vi "Layer Scan V1.vi"() -> ()   [LabVIEW 2024]
uses:
  <vilib>/DAQmx/create/channels.llb/DAQmx Create Channel (AO-Voltage-Basic).vi
  <vilib>/DAQmx/configure/timing.llb/DAQmx Timing (Sample Clock).vi
  <vilib>/DAQmx/configure/trigger.llb/DAQmx Start Trigger (Digital Edge).vi
  <vilib>/measure/NI_MAPro.lvlib
  <vilib>/express/express analysis/Spectral/XNode/ExpressSpectralMeasurementsBlockNode.xnode
  <vilib>/express/express analysis/Spectral/Block/exnSpectralBlock spectral measurements RMS poly.vi
  <vilib>/measure/NI_MABase.lvlib
  <vilib>/DAQmx/write.llb/DAQmx Write (Analog 2D DBL NChan NSamp).vi
  <vilib>/DAQmx/write.llb/DAQmx Write (Analog DBL 1Chan 1Samp).vi
  <vilib>/DAQmx/create/channels.llb/DAQmx Create Channel (AI-Voltage-Basic).vi
  <vilib>/DAQmx/write.llb/DAQmx Write (Analog 1D DBL NChan 1Samp).vi
  <vilib>/express/express analysis/Spectral/Block/exnSpectralBlock spectral measurements RMS WFM.vi
  <vilib>/DAQmx/read.llb/DAQmx Read (Analog DBL 1Chan 1Samp).vi
panel:
  out "Array":dbl[][](array[numeric])
  out "scan position #":i32
  in  "Laser Vibrometer CDAQ Channel":tag
  out "Waveform Graph":waveform(dbl)(graph)
  in  "Scan area":bool
  out "X position.":dbl
  out "Y position":dbl
  out "Galvo X Angle":dbl(graph)
  out "Galvo Y Angle":dbl(graph)
  out "time (ms)":u32
  in  "stop/save file":bool
  in  "Enable":bool=TRUE
  in  "File destination for Data":path
  out "Y MIN":dbl
  out "Y MAX":dbl
  out "X MIN":dbl
  out "X MAX":dbl
  in  "Y  voltage step(V/100)":dbl=1.0 format="%#_13g"
  in  "X  voltage step(V/100)":dbl=1.0 format="%#_13g"
  in  "offset Y":dbl format="%0.2p"
  in  "phase Y":dbl format="%.2p"
  in  "amplitude Y":dbl=1.0 format="%0.2p"
  in  "phase X":dbl format="%.2p"
  in  "amplitude X":dbl=1.0 format="%0.2p"
  in  "offset X":dbl format="%0.2p"
  out "Waveform Chart 2":waveform(dbl)(graph)
  out "Waveform Chart":waveform(dbl)(graph)
  in  "Initialize CDAQ channels":enum32{"PZT", "LV", "Galvo", "Camera"}(tab)
  in  "Pulser triggering Channel":tag
  in  "X-Axis Mirror":tag
  in  "Y-Axis Mirror":tag
  out "reference pulse":waveform(dbl)(graph)
  out "raw data":dbl[](graph)
  out "FFT":cluster{"f0":dbl, "df":dbl, "magnitude":dbl[]}(graph)
  # "Adjust Scan Area"
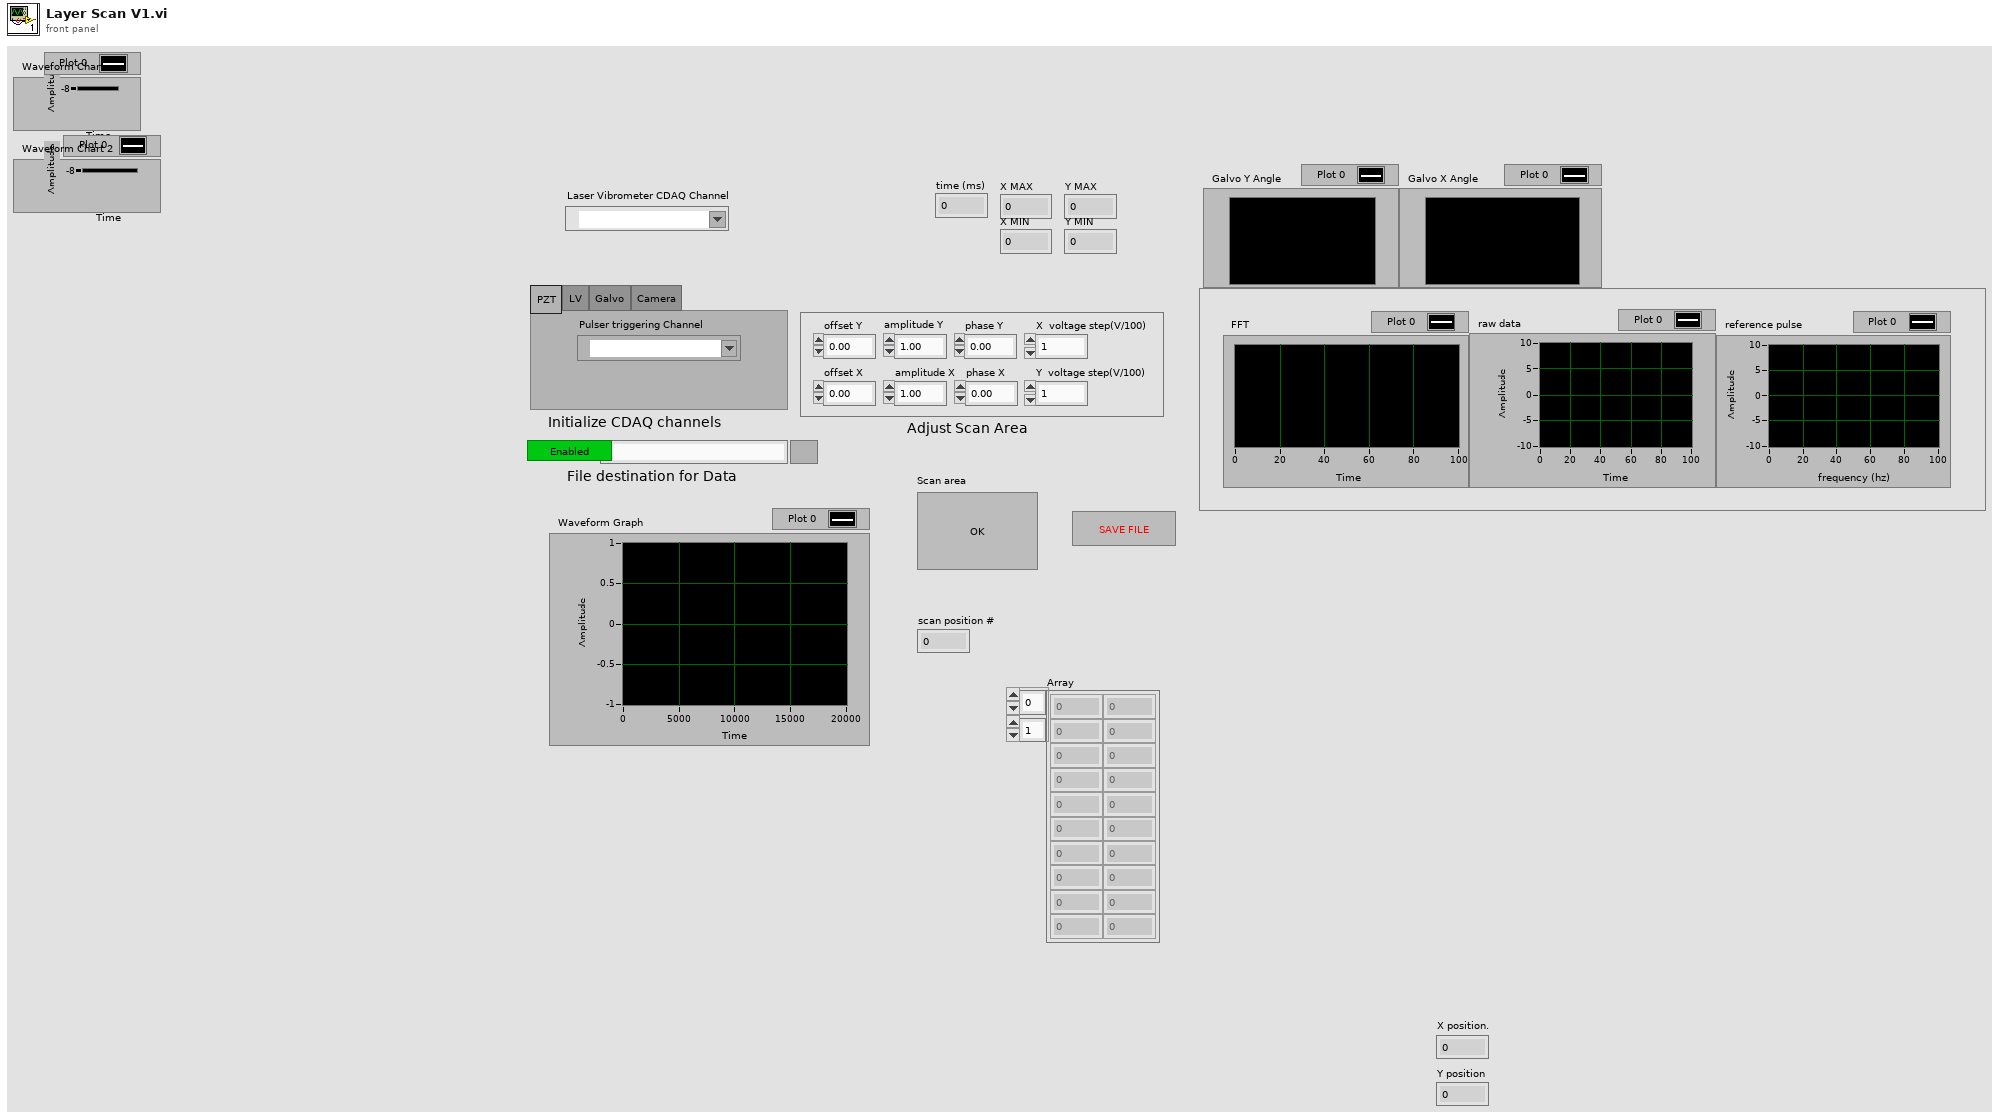
[diagram p1: front panel]
types:
  T1 = cluster{"averaging mode":u16, "weighting mode":u16, "number of averages":u32}
  T2 = cluster{"dB On (F)":bool, "unwrap phase (F)":bool, "convert to degree (F)":bool}
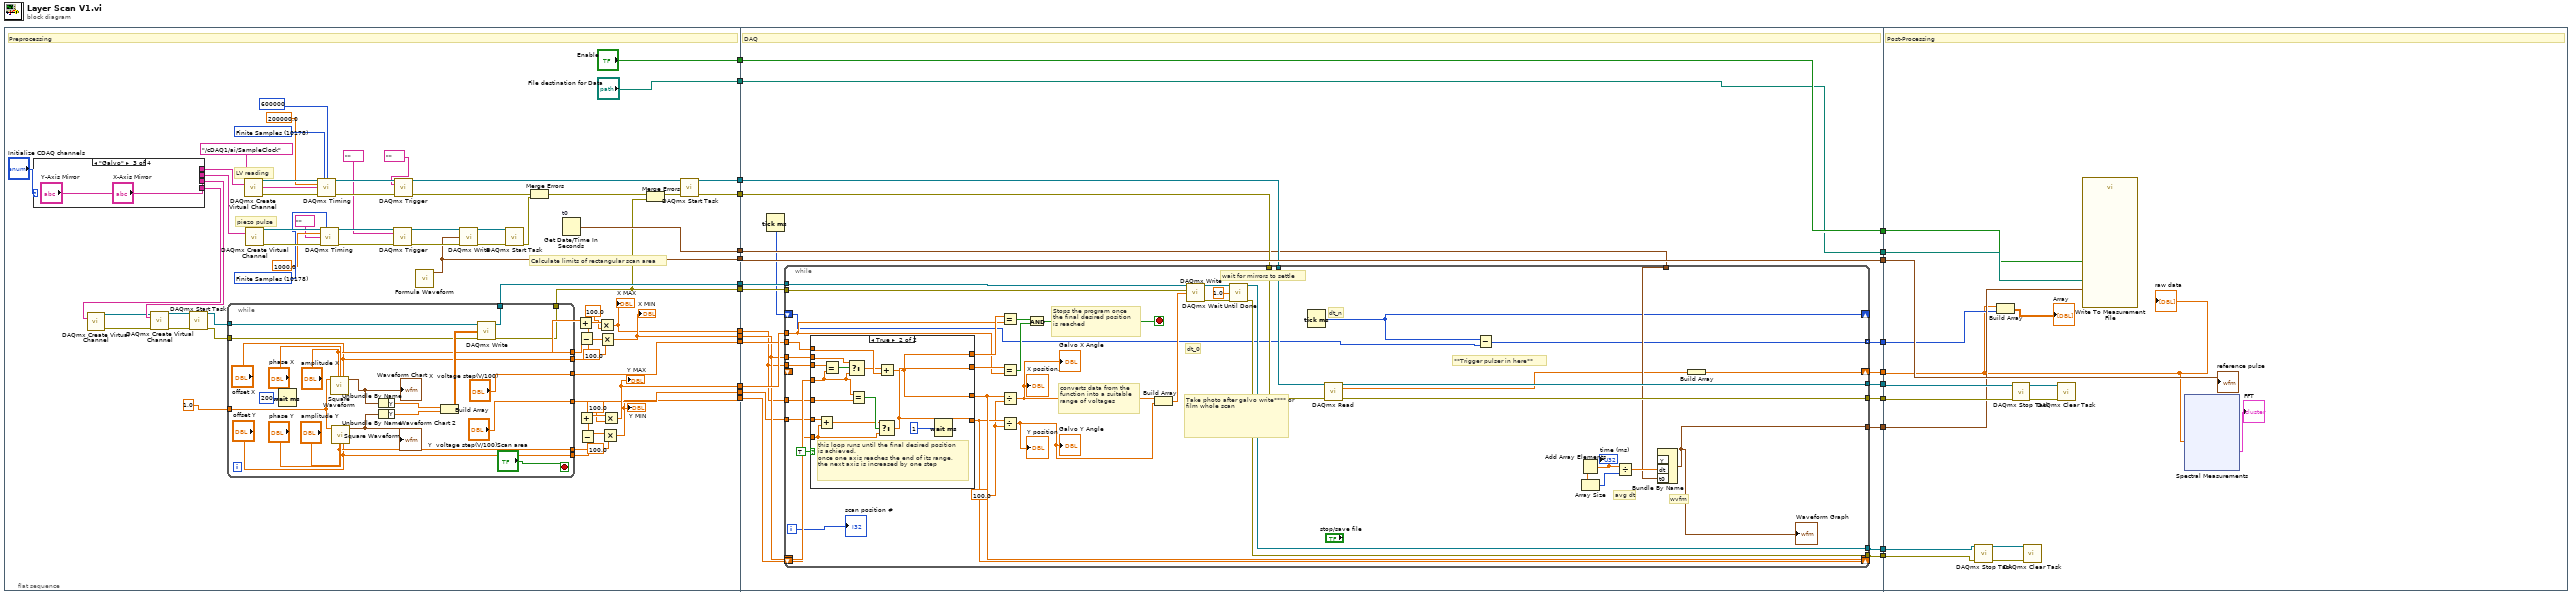
[diagram p0: block diagram]
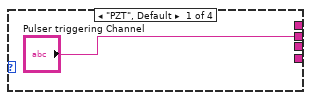
[diagram p2: hidden frame]
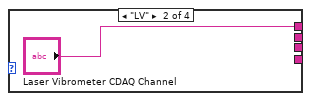
[diagram p3: hidden frame]
diagram:
  n1 = flat-sequence {
    tunnel: [w39] -> w24
    tunnel: [w38] -> w23
    tunnel: ["File destination for Data"] -> w22
    tunnel: ["Enable"] -> w21
    tunnel: [w86] -> w20
    tunnel: [w37] -> w16
    tunnel: [w36] -> w14
    tunnel: [w29] -> w13
    tunnel: [w35] -> w12
    tunnel: [w34] -> w11
    tunnel: [w33] -> w10
    tunnel: [w32] -> w9
    tunnel: [w31] -> w8
    tunnel: [w30] -> w7
    tunnel: [w125] -> w19
    tunnel: [w124] -> w18
    tunnel: w24 -> [w122]
    tunnel: w23 -> [w121]
    tunnel: w22 -> [w115]
    tunnel: w21 -> [w116]
    tunnel: w20 -> [w118]
    tunnel: [w123] -> w17
    tunnel: w16 -> [w134]
    tunnel: [w134] -> w15
    tunnel: w14 -> [w133]
    tunnel: w13 -> [w132]
    tunnel: w12 -> [w131]
    tunnel: w11 -> [w130]
    tunnel: w10 -> [w129]
    tunnel: w9 -> [w128]
    tunnel: w8 -> [w127]
    tunnel: w7 -> [w126]
    tunnel: [w120] -> w6
    tunnel: [w119] -> w5
    tunnel: [w117] -> w4
    tunnel: [w115] -> w3
    tunnel: [w116] -> w2
    tunnel: [w113] -> w1
    tunnel: w19 -> [w206]
    tunnel: w18 -> [w205]
    tunnel: w17 -> [w194]
    tunnel: w15 -> [w203]
    tunnel: w6 -> [w200]
    tunnel: w5 -> [w199]
    tunnel: w4 -> [w198]
    tunnel: w3 -> [w197]
    tunnel: w2 -> [w196]
    tunnel: w1 -> [w195]
    frame #0 {
      w45 = 10178 items=["Finite Samples"=10178, "Continuous Samples"=10123, "Hardware Timed Single Point"=12522] ("sample mode")
      w42 = 10178 items=["Finite Samples"=10178, "Continuous Samples"=10123, "Hardware Timed Single Point"=12522] ("sample mode")
      # "Calculate limits of rectangular scan area"
      # "LV reading"
      # "piezo pulse"
      # "Preprocessing"
      n2 = case shown="\"Galvo\"" "Initialize CDAQ channels" {
        tunnel: [_ "Laser Vibrometer CDAQ Channel" _ _] -> w74
        tunnel: ["Pulser triggering Channel" _ _ _] -> w75
        tunnel: [_ _ "X-Axis Mirror" _] -> w76
        tunnel: [_ _ "Y-Axis Mirror" _] -> w77
        frame "PZT", Default {
        }
        frame "LV" {
        }
        frame "Galvo" {
        }
        frame "Camera" {
        }
      }
      n3 = call-poly <vilib>:"DAQmx Create Virtual Channel.vi"("physical channels"=w77) -> ("task out"=w71:refnum<k21>, "error out"=w72:errorcluster)  [unwired: 13 in]
      n4 = call-poly <vilib>:"DAQmx Create Virtual Channel.vi"("task in"=w71, "physical channels"=w76, "error in"=w72) -> ("task out"=w69:refnum<k21>, "error out"=w70:errorcluster)  [unwired: 11 in]
      n5 = call <vilib>:"DAQmx Start Task.vi"("task/channels in"=w69, "error in"=w70) -> ("task out"=w67:refnum<k21>, "error out"=w68:errorcluster)  [unwired: 12 in]
      n6 = while {
        tunnel: w67 -> [w104]
        tunnel: w68 -> [w103]
        tunnel: ["amplitude X"] -> w84
        tunnel: ["offset X"] -> w85
        tunnel: ["amplitude Y"] -> w82
        tunnel: ["offset Y"] -> w83
        tunnel: [w98] -> w36
        tunnel: [w97] -> w29
        tunnel: ["X  voltage step(V/100)"] -> w34
        tunnel: ["Y  voltage step(V/100)"] -> w31
        tunnel: 1.0 ("frequency") -> [w93]
        stop <- "Scan area" stop-if-true
        n7 = Wait (ms)(milliseconds to wait=u32 200) -> ()  [unwired: 1 out]
        n8 = call <vilib>:"Square Waveform.vi"("offset"="offset X", "phase"="phase X", "amplitude"="amplitude X", "frequency"=w93) -> ("signal out"=w108:waveform(dbl))  [unwired: 6 in, 1 out]
        "Waveform Chart" <- w108
        n9 = call <vilib>:"Square Waveform.vi"("offset"="offset Y", "phase"="phase Y", "amplitude"="amplitude Y", "frequency"=w93) -> ("signal out"=w109:waveform(dbl))  [unwired: 6 in, 1 out]
        "Waveform Chart 2" <- w109
        n10 = Unbundle By Name(w108) -> ("Y"=w107:dbl[])
        n11 = Unbundle By Name(w109) -> ("Y"=w106:dbl[])
        n12 = Build Array(w107, w106) -> (w105:dbl[][])
        n13 = call-poly <vilib>:"DAQmx Write.vi"("task/channels in"=w104, "data"=w105, "error in"=w103) -> ("task out"=w98:refnum<k21>, "error out"=w97:errorcluster)  [unwired: 10 in, 1 out]
      }
      n14 = call-poly <vilib>:"DAQmx Create Virtual Channel.vi"("physical channels"=w74) -> ("task out"=w52:refnum<k21>, "error out"=w53:errorcluster)  [unwired: 13 in]
      n15 = call-poly <vilib>:"DAQmx Create Virtual Channel.vi"("physical channels"=w75) -> ("task out"=w57:refnum<k21>, "error out"=w58:errorcluster)  [unwired: 13 in]
      n16 = call-poly <vilib>:"DAQmx Timing.vi"("task/channels in"=w52, "sample mode"=w42, "samples per channel"=600000, "rate"=200000.0, "source"=tag "/cDAQ1/ai/SampleClock", "error in"=w53) -> ("task out"=w54:refnum<k21>, "error out"=w55:errorcluster)  [unwired: 8 in]
      n17 = call-poly <vilib>:"DAQmx Timing.vi"("task/channels in"=w57, "sample mode"=w45, "rate"=1000.0, "source"=tag "", "error in"=w58) -> ("task out"=w59:refnum<k21>, "error out"=w60:errorcluster)  [unwired: 9 in]
      n18 = call-poly <vilib>:"DAQmx Trigger.vi"("task/channels in"=w59, "source"=tag "", "error in"=w60) -> ("task out"=w61:refnum<k21>, "error out"=w62:errorcluster)  [unwired: 11 in]
      n19 = call-poly <vilib>:"DAQmx Trigger.vi"("task/channels in"=w54, "source"=tag "", "error in"=w55) -> ("task out"=w56:refnum<k21>, "error out"=w66:errorcluster)  [unwired: 11 in]
      n20 = call <vilib>:"Formula Waveform.vi"() -> ("signal out"=w37:waveform(dbl))  [unwired: 10 in, 1 out]
      n21 = call-poly <vilib>:"DAQmx Write.vi"("task/channels in"=w61, "data"=w37, "error in"=w62) -> ("task out"=w63:refnum<k21>, "error out"=w64:errorcluster)  [unwired: 10 in, 1 out]
      n22 = call <vilib>:"DAQmx Start Task.vi"("task/channels in"=w63, "error in"=w64) -> ("error out"=w65:errorcluster)  [unwired: 12 in, 1 out]
      n23 = Merge Errors(w66, w65) -> (w28:errorcluster)
      n24 = Get Date/Time In Seconds "t0"() -> (seconds since 1Jan1904=w86:timestamp)
      n25 = Add(x=w84, y=w85) -> (x+y=w80:dbl)
      n26 = Subtract(x=w85, y=w84) -> (x-y=w78:dbl)
      n27 = Add(x=w82, y=w83) -> (x+y=w81:dbl)
      n28 = Subtract(x=w83, y=w82) -> (x-y=w79:dbl)
      n29 = Multiply(x=w80, y=100.0) -> (x*y=w32:dbl)
      "X MAX" <- w32
      n30 = Multiply(x=w78, y=100.0) -> (x*y=w33:dbl)
      "X MIN" <- w33
      n31 = Multiply(x=w79, y=100.0) -> (x*y=w30:dbl)
      "Y MIN" <- w30
      n32 = Multiply(x=w81, y=100.0) -> (x*y=w35:dbl)
      "Y MAX" <- w35
      n33 = Merge Errors(w28, w29) -> (w27:errorcluster)
      n34 = call <vilib>:"DAQmx Start Task.vi"("task/channels in"=w56, "error in"=w27) -> ("task out"=w39:refnum<k21>, "error out"=w38:errorcluster)  [unwired: 12 in]
    }
    frame #1 {
      # "DAQ"
      n35 = Tick Count (ms)() -> (millisecond timer value=w114:u32)
      n36 = while {
        shift-right: [w171] -> _
        shift-left: w129 -> [w178]
        shift-right: [w170] -> _
        shift-left: w126 -> [w177]
        tunnel: w133 -> [w165]
        tunnel: w132 -> [w164]
        tunnel: w127 -> [w163]
        tunnel: w130 -> [w162]
        tunnel: w128 -> [w161]
        tunnel: w128 -> [w160]
        tunnel: w131 -> [w159]
        tunnel: w129 -> [w158]
        tunnel: [w154] -> w125
        tunnel: [w153] -> w124
        tunnel: w122 -> [w152]
        tunnel: w121 -> [w151]
        tunnel: [w150] -> w120
        tunnel: [w149] -> w119
        tunnel: w118 -> [w145]
        tunnel: [w142] -> w117
        shift-right: [w139] -> _
        shift-left: w114 -> [w138]
        shift-right: [w137] -> w123
        shift-left: _ -> [_]
        tunnel: [w135] -> w113 mode=indexing
        i -> [w141]
        stop <- w174 stop-if-true
        w169 = 100.0 ("x")
        # "dt_n"
        # "**Trigger pulser in here**"
        # "wvfm"
        # "avg dt"
        # "wait for mirrors to settle"
        # "dt_0"
        # "Take photo after galvo write**** or film whole scan"
        # "converts data from the\nfunction into a suitable \nrange of voltages"
        # "Stops the program once\nthe final desired position \nis reached"
        n37 = case shown="True" TRUE {
          tunnel: w178 -> [_ w179]
          tunnel: [_ w187] -> w171
          tunnel: w177 -> [_ w189]
          tunnel: [_ w188] -> w170
          tunnel: [_ w187] -> w173
          tunnel: [_ w188] -> w172
          tunnel: w163 -> [_ w185]
          tunnel: w162 -> [_ w184]
          tunnel: w161 -> [_ w183]
          tunnel: w160 -> [_ w182]
          tunnel: w158 -> [_ w181]
          frame False {
          }
          frame True {
            # "this loop runs until the final desired position\nis achieved.\nonce one axis reaches the end of its range,\nthe next axis is increased by one step"
            n38 = Add(x=w185, y=w189) -> (x+y=w190:dbl)
            n39 = Equal?(x=w183, y=w179) -> (x = y?=w192:bool)
            n40 = Select(t=w181, s=w192, f=w179) -> (s? t:f=w180:dbl)
            n41 = Equal?(x=w179, y=w182) -> (x = y?=w191:bool)
            n42 = Select(t=w190, s=w191, f=w189) -> (s? t:f=w188:dbl)
            n43 = Add(x=w180, y=w184) -> (x+y=w187:dbl)
            n44 = Wait (ms)(milliseconds to wait=u32 1) -> ()  [unwired: 1 out]
          }
        }
        n45 = Equal?(x=w173, y=w159) -> (x = y?=w176:bool)
        n46 = Equal?(x=w172, y=w159) -> (x = y?=w175:bool)
        n47 = Divide(x=w171, y=w169) -> (x/y=w167:dbl)
        "X position." <- w167
        "Galvo X Angle" <- w167
        n48 = Divide(x=w170, y=w169) -> (x/y=w168:dbl)
        "Y position" <- w168
        "Galvo Y Angle" <- w168
        n49 = And(x=w176, y=w175) -> (x .and. y?=w174:bool)
        n50 = Build Array(w167, w168) -> (w166:dbl[])
        n51 = call-poly <vilib>:"DAQmx Write.vi"("task/channels in"=w165, "data"=w166, "error in"=w164) -> ("task out"=w157:refnum<k21>, "error out"=w156:errorcluster)  [unwired: 10 in, 1 out]
        n52 = call <vilib>:"DAQmx Wait Until Done.vi"("task/channels in"=w157, "timeout (sec)"=1.0, "error in"=w156) -> ("task out"=w150:refnum<k21>, "error out"=w149:errorcluster)  [unwired: 11 in]
        n53 = Tick Count (ms)() -> (millisecond timer value=w139:u32)
        n54 = call-poly <vilib>:"DAQmx Read.vi"("task/channels in"=w152, "error in"=w151) -> ("task out"=w154:refnum<k21>, "data"=w144:dbl, "error out"=w153:errorcluster)  [unwired: 11 in]
        n55 = Subtract(x=w139, y=w138) -> (x-y=w135:u32)
        n56 = Array Size() -> (array=w136:dbl[], size(s)=w147:i32)
        n57 = Add Array Elements(numeric array=w136) -> (sum=w146:dbl)
        "time (ms)" <- w146
        n58 = Divide(x=w146, y=w147) -> (x/y=w148:dbl)
        n59 = Bundle By Name("dt"=w148, "t0"=w145) -> (w142:waveform(dbl))  [unwired: 2 in]
        "Waveform Graph" <- w142
        n60 = Build Array(w144) -> (w137:dbl[])
        "scan position #" <- w141
      }
    }
    frame #2 {
      # "Post-Processing"
      n61 = call <vilib>:"DAQmx Stop Task.vi"("task/channels in"=w200, "error in"=w199) -> ("task out"=w201:refnum<k21>, "error out"=w202:errorcluster)  [unwired: 12 in]
      n62 = Build Array(w194, w195) -> (→"Array":dbl[][])
      n63 = call <vilib>:"DAQmx Stop Task.vi"("task/channels in"=w206, "error in"=w205) -> ("task out"=w207:refnum<k21>, "error out"=w208:errorcluster)  [unwired: 12 in]
      n64 = call <vilib>:"DAQmx Clear Task.vi"("task in"=w201, "error in"=w202) -> ()  [unwired: 13 in, 1 out]
      n65 = call <vilib>:"DAQmx Clear Task.vi"("task in"=w207, "error in"=w208) -> ()  [unwired: 13 in, 1 out]
      n66 = call "Write To Measurement File"("Signals"=w198, "Enable"=w196, "Filename"=w197) -> ()  [unwired: 14 in, 3 out]
      n67 = xnode "Spectral Measurements"("Signals"=w194) -> ("FFT - (RMS)"=→"FFT":cluster{"f0":dbl, "df":dbl, "magnitude":dbl[]})  [unwired: 1 in, 2 out]
      "raw data" <- w194
      "reference pulse" <- w203
    }
  }
